vi "serialization tests.vi"() -> ()   [LabVIEW 2013, in "user code tests.lvlib"]
uses:
  user code tests.lvlib
  module/configuration/user tag bus module configuration.lvclass
panel:
  out "classes equal":bool
  out "no error":errorcluster
  out "no error":errorcluster
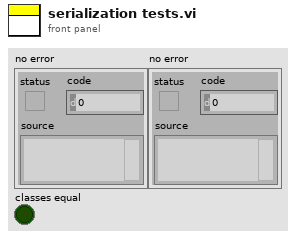
[diagram p1: front panel]
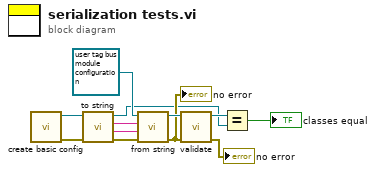
[diagram p0: block diagram]
diagram:
  n1 = call "create basic config.vi"() -> ("error out"=w4:errorcluster, "user tag bus module configuration out"=w3:refnum<class "user tag bus module configuration.lvclass">)  [unwired: 8 in, 2 out]
  n2 = call-dynamic "to string.vi"("error in"=w4, "user tag bus module configuration In"=w3) -> ("error out"=w12:errorcluster, "data"=w11:string, "version"=w10:string, "user tag bus module configuration Out"=w1:refnum<class "user tag bus module configuration.lvclass">)  [unwired: 6 in]
  n3 = call-dynamic "from string.vi"("error in"=w12, "data"=w11, "version"=w10, "user tag bus module configuration In"=refnum<class "user tag bus module configuration.lvclass"> refnum ("tag bus configurable plugin module configuration")) -> ("error out"=w7:errorcluster, "user tag bus module configuration Out"=w9:refnum<class "user tag bus module configuration.lvclass">)  [unwired: 6 in]
  "no error" <- w7
  n4 = call-dynamic "validate.vi"("error in"=w7, "tag bus configurable plugin module configuration in"=w9) -> ("error out"=→"no error":errorcluster, "tag bus configurable plugin module configuration out"=w2:refnum<class "user tag bus module configuration.lvclass">)  [unwired: 8 in]
  n5 = Equal?(x=w2, y=w1) -> (x = y?=→"classes equal":bool)
